vi "New-ExitCoords.vi"(4 "LUT in":dbl[][](array[numeric]), 5 "correction trial":bool, 6 "Trials":i32[](array[numeric]), 7 "Blue/Yellow":bool, 8 "exit rad":dbl, 9 "hab rad":dbl, 10 "centroid":dbl[](array[numeric]), 11 "center":dbl[](array[numeric])) -> (0 "LUT out":dbl[][](array[numeric]), 1 "output cluster 2":T1, 2 "CW/CCW":bool, 3 "output cluster":T2)   [LabVIEW 2019]
uses:
  <vilib>/Analysis/baseanly.llb/Real A x B.vi
  <vilib>/Analysis/Matrix/Numeric/Conversions/Array To Matrix - RA.vi
  <vilib>/Analysis/Matrix/Numeric/Conversions/Matrix To Array - RM.vi
  <vilib>/Analysis/NI_AALBase.lvlib
  <vilib>/Analysis/Matrix/NI_Matrix.lvlib
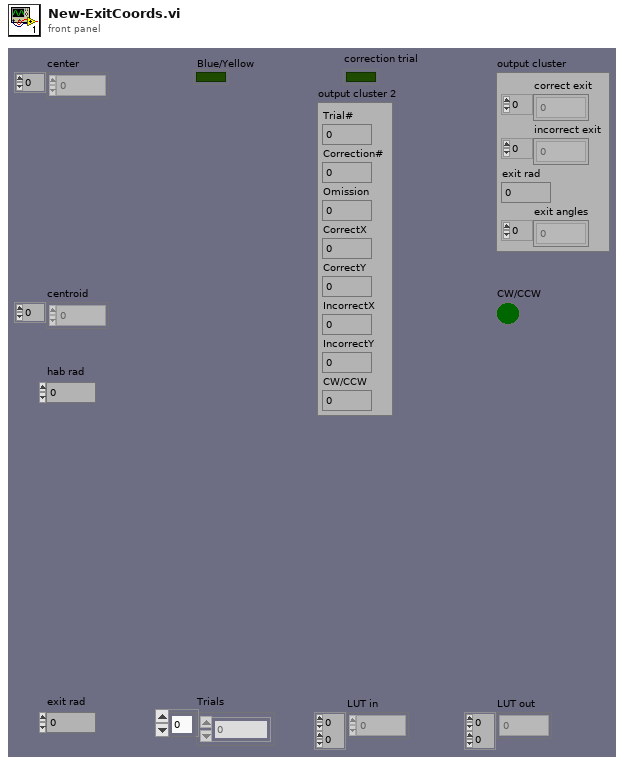
[diagram p1: front panel]
types:
  T1 = cluster{"Trial#":dbl, "Correction#":dbl, "Omission":dbl, "CorrectX":dbl, "CorrectY":dbl, "IncorrectX":dbl, "IncorrectY":dbl, "CW/CCW":dbl}
  T2 = cluster{"correct exit":dbl[], "incorrect exit":dbl[], "exit rad":dbl, "exit angles":dbl[]}
  T3 = typedef "NI_Matrix.lvlib/RealMatrix.ctl" = dbl[][]
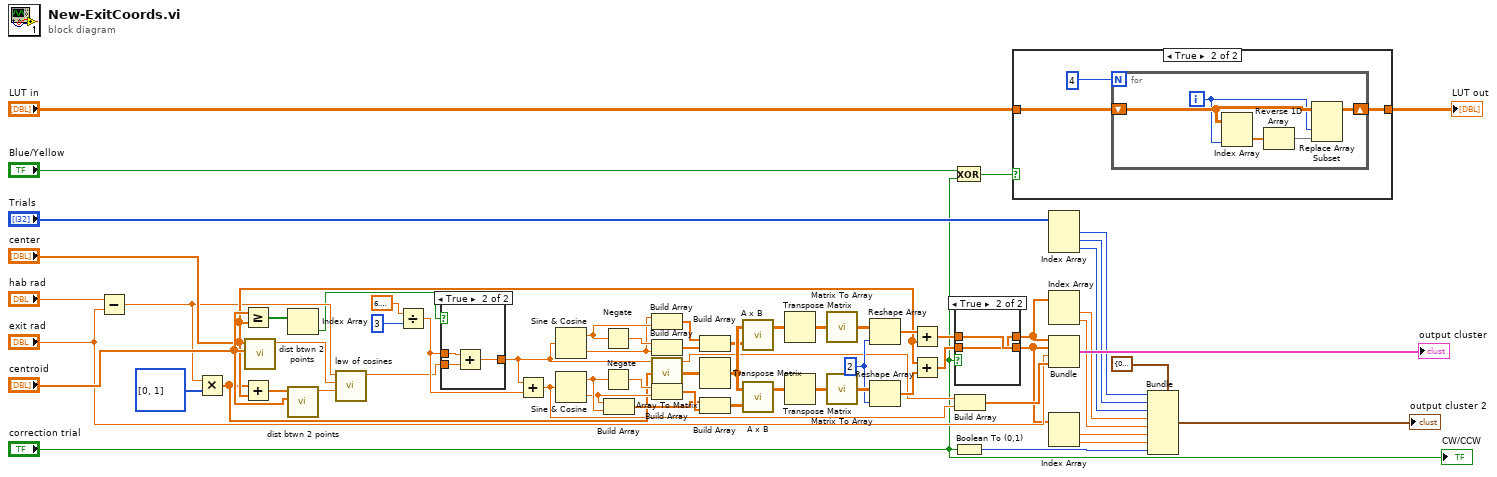
[diagram p0: block diagram]
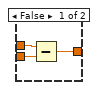
[diagram p4: hidden frame]
diagram:
  w30 = u32 2 ("y")
  n1 = Subtract(x="hab rad", y="exit rad") -> (x-y=w28:dbl)
  n2 = Multiply(x=w28, y=i32[] [0, 1]) -> (x*y=w31:dbl[])
  n3 = Greater Or Equal?(x="centroid", y="center") -> (x >= y?=w27:bool[])
  n4 = Add(x=w31, y="center") -> (x+y=w59:dbl[])
  n5 = call "dist btwn 2 points.vi"("coord pair 2"="centroid", "coord pair1"="center") -> ("dist"=w45:dbl)  [unwired: 9 in]
  n6 = Index Array(array=w27) -> (element=w21:bool)  [unwired: 1 in]
  n7 = call "dist btwn 2 points.vi"("coord pair 2"="centroid", "coord pair1"=w59) -> ("dist"=w46:dbl)  [unwired: 9 in]
  n8 = call "law of cosines.vi"("target to exit dist"=w46, "center to target dist"=w45, "center to exit dist"=w28) -> ("angle"=w25:dbl)  [unwired: 8 in]
  n9 = Divide(x=6.283185307179586, y=3) -> (x/y=w26:dbl)
  n10 = case shown="True" w21 {
    tunnel: w26 -> [w66 w67]
    tunnel: w25 -> [w65 w69]
    tunnel: [w64 w68] -> w23
    frame False {
      n11 = Subtract(x=w66, y=w65) -> (x-y=w64:dbl)
    }
    frame True {
      n12 = Add(x=w67, y=w69) -> (x+y=w68:dbl)
    }
  }
  n13 = Add(x=w23, y=w26) -> (x+y=w24:dbl)
  n14 = Sine & Cosine(0:w23) -> (1:w38:dbl, 2:w37:dbl)
  n15 = Sine & Cosine(0:w24) -> (1:w48:dbl, 2:w47:dbl)
  n16 = Negate(x=w38) -> (-x=w39:dbl)
  n17 = Negate(x=w48) -> (-x=w49:dbl)
  n18 = Build Array(w47, w48) -> (w50:dbl[])
  n19 = Build Array(w37, w38) -> (w40:dbl[])
  n20 = Build Array(w39, w37) -> (w41:dbl[])
  n21 = call-poly <vilib>:"Array To Matrix.vi"("Real 1D Array"=w31) -> ("Real Matrix (Column Vector)"=w60:T3)
  n22 = Build Array(w49, w47) -> (w51:dbl[])
  n23 = Build Array ("Build Matrix")(w40, w41) -> (w42:T3)
  n24 = Transpose Matrix(1:w60) -> (0:w61:T3)
  n25 = Build Array ("Build Matrix")(w50, w51) -> (w52:T3)
  n26 = call-poly <vilib>:"A x B.vi"("B"=w42, "A"=w61) -> ("A x B"=w57:T3)  [unwired: 1 out]
  n27 = call-poly <vilib>:"A x B.vi"("B"=w52, "A"=w61) -> ("A x B"=w58:T3)  [unwired: 1 out]
  n28 = Transpose Matrix(1:w57) -> (0:w54:T3)
  n29 = Transpose Matrix(1:w58) -> (0:w56:T3)
  n30 = call-poly <vilib>:"Matrix To Array.vi"("Real Matrix"=w54) -> ("Real 2D Array"=w53:dbl[][])
  n31 = call-poly <vilib>:"Matrix To Array.vi"("Real Matrix"=w56) -> ("Real 2D Array"=w55:dbl[][])
  n32 = Reshape Array(w53, w30) -> (w35:dbl[])
  n33 = Reshape Array(w55, w30) -> (w34:dbl[])
  n34 = Add(x=w35, y="center") -> (x+y=w20:dbl[])
  n35 = Add(x="center", y=w34) -> (x+y=w19:dbl[])
  n36 = Exclusive Or(1:"correction trial", 2:"Blue/Yellow") -> (0:w14:bool)
  n37 = Boolean To (0,1)(Boolean="correction trial") -> (0, 1=w10:i16)
  n38 = case shown="True" "correction trial" {
    tunnel: w20 -> [w71 w73]
    tunnel: [w71 w72] -> w13
    tunnel: w19 -> [w70 w72]
    tunnel: [w70 w73] -> w12
    frame False {
    }
    frame True {
    }
  }
  n39 = Build Array(w23, w24) -> (w29:dbl[])
  n40 = case shown="True" w14 {
    tunnel: "LUT in" -> [w74 w77]
    tunnel: [w74 w75] -> w15
    frame False {
    }
    frame True {
      n41 = for {
        N: 4 -> [_]
        shift-right: [w78] -> w75
        shift-left: w77 -> [w80]
        i -> [w79]
        n42 = Index Array(array=w80, index (col)=w79) -> (element=w82:dbl[])  [unwired: 1 in]
        n43 = Reverse 1D Array(array=w82) -> (reversed array=w81:dbl[])
        n44 = Replace Array Subset(array=w80, new element=w81, index (col)=w79) -> (w78:dbl[][])  [unwired: 1 in]
      }
    }
  }
  "LUT out" <- w15
  n45 = Index Array(array="Trials") -> (element #1=w4:i32, element #2=w5:i32, element #3=w1:i32)  [unwired: 3 in]
  n46 = Index Array(array=w13) -> (element #1=w6:dbl, element #2=w7:dbl)  [unwired: 2 in]
  n47 = Bundle(w13, w12, "exit rad"="exit rad", w29) -> (→"output cluster":cluster{dbl[], dbl[], "exit rad":dbl, dbl[]})  [unwired: 1 in]
  n48 = Index Array(array=w12) -> (element #1=w8:dbl, element #2=w9:dbl)  [unwired: 2 in]
  n49 = Bundle(cluster=T1 {"Trial#"=0.0, "Correction#"=0.0, "Omission"=0.0, "CorrectX"=0.0, "CorrectY"=0.0, "IncorrectX"=0.0, "IncorrectY"=0.0, "CW/CCW"=0.0}, "Trial#"=w4, "Correction#"=w5, "Omission"=w1, "CorrectX"=w6, "CorrectY"=w7, "IncorrectX"=w8, "IncorrectY"=w9, "CW/CCW"=w10) -> (→"output cluster 2":T1)
  "CW/CCW" <- "correction trial"
